vi "Set Splitter Possition.vi"(4 "Hidden position":i32=2, 6 "Visible position":i32=22, 8 "Add(t)":bool, 9 "Visible":bool, 10 "Splitter Reference":refnum<vi>, 11 "Splitter to Modify":refnum<vi>) -> (0 "error out":errorcluster)   [LabVIEW 2020, in "Panther Dashboard.lvlib"]
uses:
  Panther Dashboard.lvlib
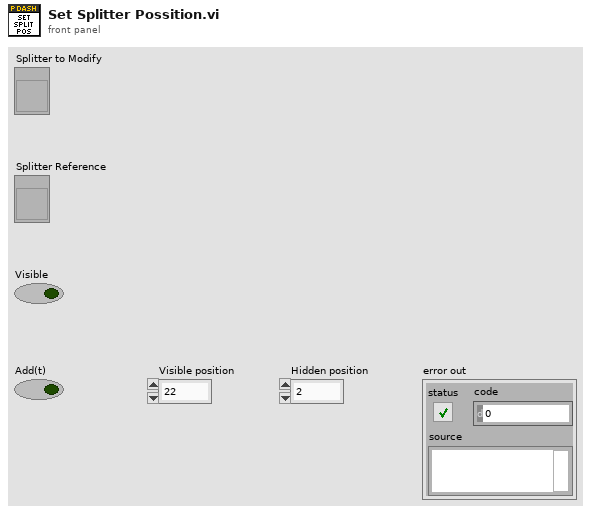
[diagram p1: front panel]
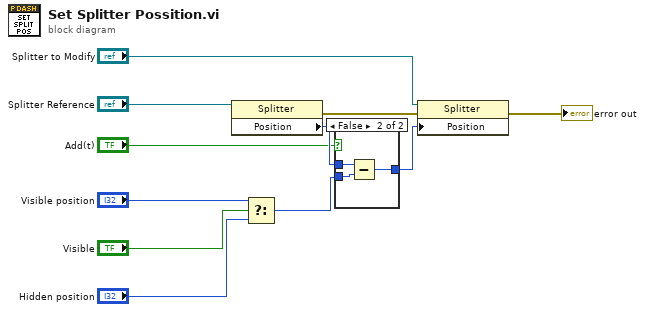
[diagram p0: block diagram]
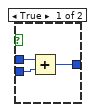
[diagram p2: hidden frame]
diagram:
  n1 = property class="Splitter"(reference="Splitter Reference") -> (error out=w11:errorcluster, "Position"=w9:i32)  [unwired: 1 in, 1 out]
  n2 = Select(t="Visible position", s="Visible", f="Hidden position") -> (s? t:f=w5:i32)
  n3 = case shown="False" "Add(t)" {
    tunnel: w9 -> [w14 w17]
    tunnel: w5 -> [w13 w16]
    tunnel: [w12 w15] -> w1
    frame True {
      n4 = Add(x=w14, y=w13) -> (x+y=w12:i32)
    }
    frame False {
      n5 = Subtract(x=w17, y=w16) -> (x-y=w15:i32)
    }
  }
  n6 = property class="Splitter"(reference="Splitter to Modify", error in=w11, "Position"=w1) -> (error out=→"error out":errorcluster)  [unwired: 1 out]
